vi "Check sensor str.vi"(7 "error in (no error)":errorcluster, 9 "Sensor value in":dbl, 10 "string":string) -> (0 "error out":errorcluster, 2 "Sensor value out":dbl)   [LabVIEW 2020, in "Control de MaP.lvlib"]
uses:
  Control de MaP.lvlib
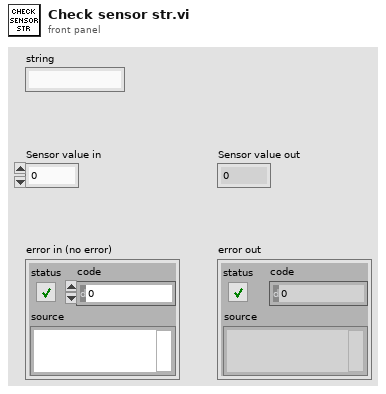
[diagram p1: front panel]
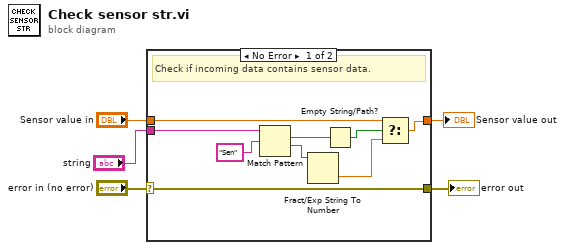
[diagram p0: block diagram]
diagram:
  n1 = case shown="No Error" "error in (no error)" {
    selector: "error in (no error)" -> [w7 w15]
    tunnel: [w14 w16] -> w5
    tunnel: "Sensor value in" -> [w11 w16]
    tunnel: [w7 w15] -> w2
    tunnel: "string" -> [w6 _]
    frame No Error {
      # "Check if incoming data contains sensor data."
      n2 = Match Pattern(string=w6, regular expression="Sen") -> (match substring=w9:string, after substring=w12:string)  [unwired: 1 in, 2 out]
      n3 = Fract/Exp String To Number(string=w12) -> (number=w13:dbl)  [unwired: 3 in, 1 out]
      n4 = Empty String/Path?(string/path=w9) -> (empty?=w10:bool)
      n5 = Select(t=w11, s=w10, f=w13) -> (s? t:f=w14:dbl)
    }
    frame Error {
    }
  }
  "Sensor value out" <- w5
  "error out" <- w2
